vi "Asylum_WriteValue.vi"(8 "error in (no error)":errorcluster, 9 "value":dbl, 10 "parameterName":string, 11 "Application":refnum<k7>) -> (0 "error out":errorcluster, 3 "Application":refnum<k7>)   [LabVIEW 2016]
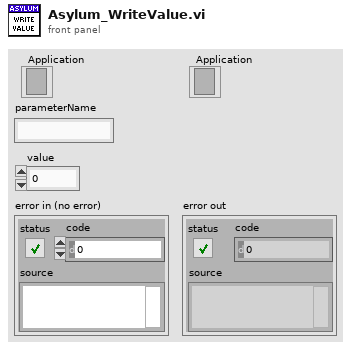
[diagram p1: front panel]
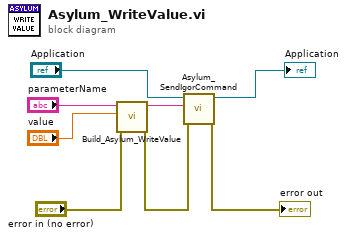
[diagram p0: block diagram]
diagram:
  n1 = call "Build_Asylum_WriteValue.vi"("error in (no error)"="error in (no error)", "value"="value", "parameterName"="parameterName") -> ("error out"=w3:errorcluster, "Command"=w8:string)  [unwired: 7 in]
  n2 = call "Asylum_SendIgorCommand.vi"("error in (no error)"=w3, "command"=w8, "Application"="Application") -> ("error out"=→"error out":errorcluster, "Application"=→"Application":refnum<k7>)  [unwired: 5 in, 2 out]
